vi "LockBit_NB_Core_DDR.vi"(11 "error in (no error)":errorcluster) -> (2 "NB Lock Bit":bool, 3 "DDR Lock Bit":bool, 4 "Core0 Lock Bit":bool, 6 "Core1 Lock Bit":bool, 8 "Core2 Lock Bit":bool, 10 "Core3 Lock Bit":bool, 15 "error out":errorcluster)   [LabVIEW 2011]
doc: "This VI reads the lock bit state for the Core, NB, and DDR PLL's.\n\nOutputs:\n1. NB/Core0-3/DDR Lock Result: The lock bit result for each PLL (1 locked or 0 unlocked)."
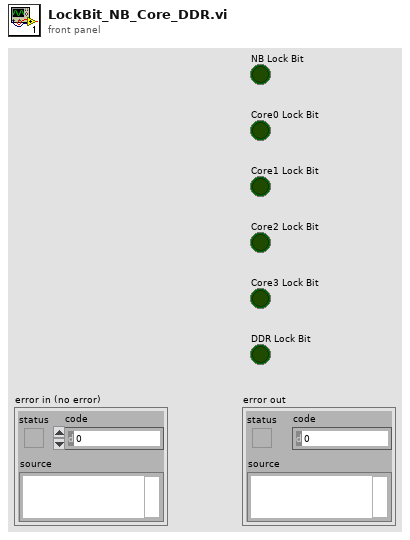
[diagram p1: front panel]
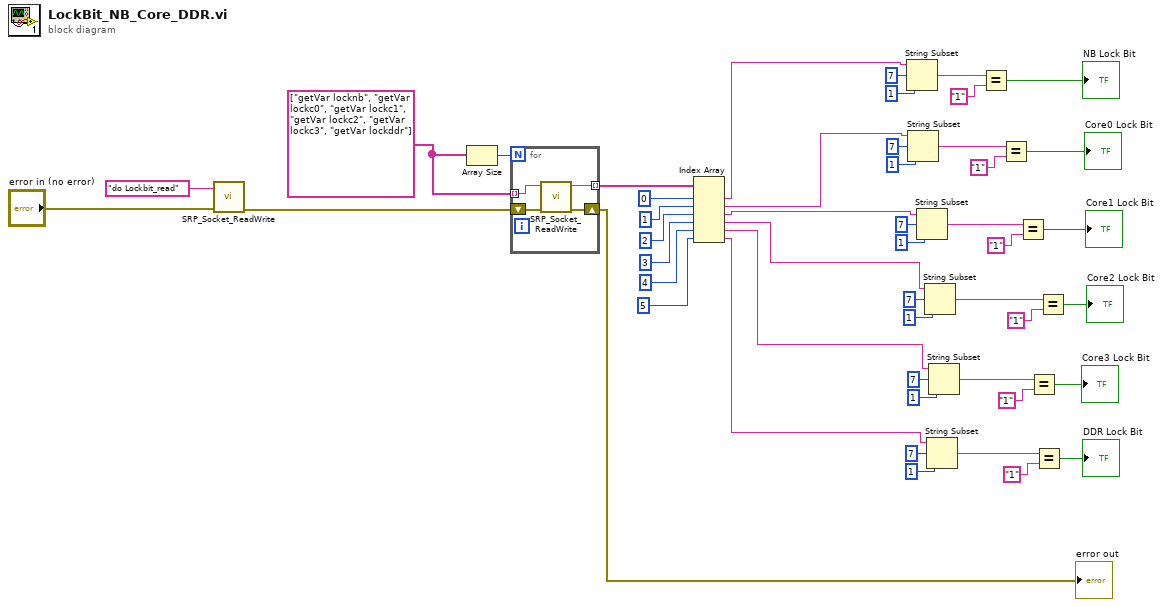
[diagram p0: block diagram]
diagram:
  w45 = string[] ["getVar locknb", "getVar lockc0", "getVar lockc1", "getVar lockc2", "getVar lockc3", "getVar lockddr"]
  n1 = call "SRP_Socket_ReadWrite.vi"("error in (no error)"="error in (no error)", "Data In"="do Lockbit_read") -> ("error out"=w46:errorcluster)  [unwired: 7 in, 1 out]
  n2 = Array Size(array=w45) -> (size(s)=w47:i32)
  n3 = for {
    N: w47 -> [_]
    shift-right: [w52] -> w37
    shift-left: w46 -> [w53]
    tunnel: w45 -> [w51] mode=indexing
    tunnel: [w50] -> w44 mode=indexing
    n4 = call "SRP_Socket_ReadWrite.vi"("error in (no error)"=w53, "Data In"=w51) -> ("error out"=w52:errorcluster, "Data Out"=w50:string)  [unwired: 7 in]
  }
  "error out" <- w37
  n5 = Index Array(array=w44, index #1=0 ("index"), index #2=1 ("index"), index #3=2 ("index"), index #4=3 ("index"), index #5=4 ("index"), index #6=5 ("index")) -> (element #1=w34:string, element #2=w23:string, element #3=w22:string, element #4=w21:string, element #5=w20:string, element #6=w19:string)
  n6 = String Subset(string=w34, offset (0)=7, length (rest)=1 ("length (rest)")) -> (substring=w17:string)
  n7 = String Subset(string=w23, offset (0)=7, length (rest)=1 ("length (rest)")) -> (substring=w6:string)
  n8 = String Subset(string=w22, offset (0)=7, length (rest)=1 ("length (rest)")) -> (substring=w7:string)
  n9 = String Subset(string=w21, offset (0)=7, length (rest)=1 ("length (rest)")) -> (substring=w8:string)
  n10 = String Subset(string=w19, offset (0)=7, length (rest)=1 ("length (rest)")) -> (substring=w10:string)
  n11 = String Subset(string=w20, offset (0)=7, length (rest)=1 ("length (rest)")) -> (substring=w9:string)
  n12 = Equal?(x=w17, y="1") -> (x = y?=→"NB Lock Bit":bool)
  n13 = Equal?(x=w6, y="1") -> (x = y?=→"Core0 Lock Bit":bool)
  n14 = Equal?(x=w7, y="1") -> (x = y?=→"Core1 Lock Bit":bool)
  n15 = Equal?(x=w9, y="1") -> (x = y?=→"Core3 Lock Bit":bool)
  n16 = Equal?(x=w10, y="1") -> (x = y?=→"DDR Lock Bit":bool)
  n17 = Equal?(x=w8, y="1") -> (x = y?=→"Core2 Lock Bit":bool)
